vi "Exit.vi"(8 "error in (no error)":errorcluster, 11 "Old State":refnum<class "State.lvclass">) -> (0 "error out":errorcluster, 3 "New State":refnum<class "State.lvclass">)   [LabVIEW 2024, in "State.lvlib" / "State.lvclass"]
doc: "This is an abstract method. Override this method to define the behavior when you leave the state."
uses:
  State.lvclass
  State.lvclass/State.ctl
  <vilib>/NI/Actors/State Actor/State Actor/State Actor.lvclass
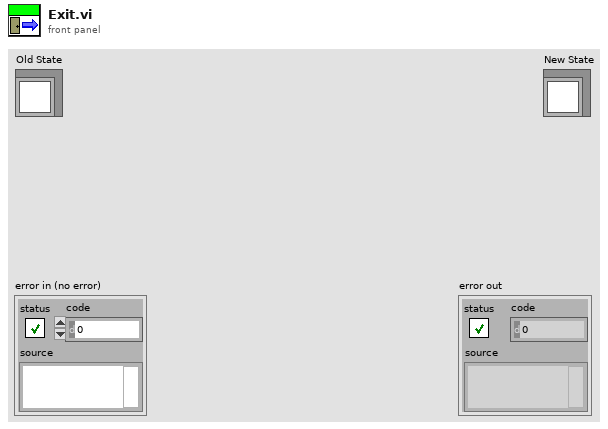
[diagram p1: front panel]
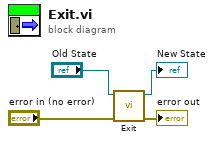
[diagram p0: block diagram]
diagram:
  n1 = call-parent "Exit.vi"("error in (no error)"="error in (no error)", "Old State"="Old State") -> ("error out"=→"error out":errorcluster, "New State"=→"New State":refnum<class "State.lvclass">)  [unwired: 8 in]
